vi "Error Handler.vi"(8 "error in (no error)":errorcluster, 9 "Error State":i32, 10 "Ignore Errors (Runtime)":i32[](array[numeric]), 11 "Queue In":refnum<queue>) -> (0 "dup error in":errorcluster, 3 "Queue Out":refnum<queue>)   [LabVIEW 2020, in "Enum Queue State Machine.lvlib"]
doc: "Process an error that occurred in the Event Handling Loop, either by ignoring it, or generating an \"Error\" message."
uses:
  Enum Queue State Machine.lvlib
  Controls/Enum Message.ctl
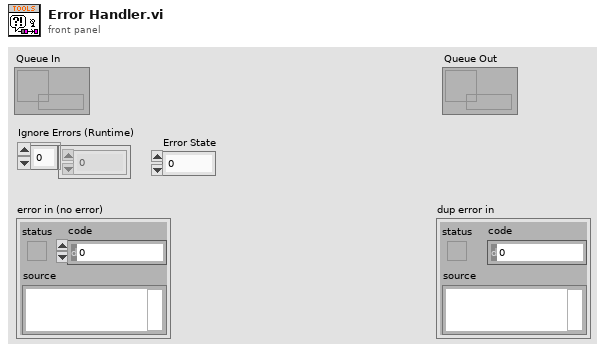
[diagram p1: front panel]
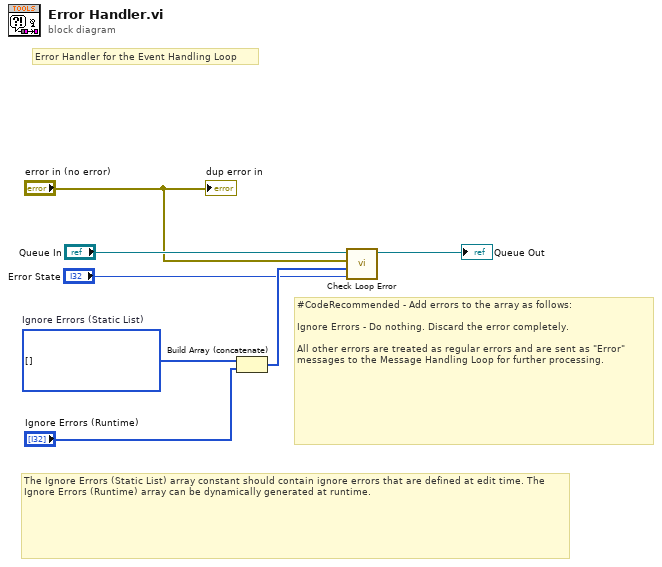
[diagram p0: block diagram]
diagram:
  w7 = i32[] []  # Ignore Errors (Static List)
  # "The Ignore Errors (Static List) array constant should contain ignore errors that are defined at edit time. The Ignore Errors (Runtime) array can be dynamically generated at runtime."
  # "#CodeRecommended - Add errors to the array as follows:\n\nIgnore Errors - Do nothing. Discard the error completely.\n\nAll other errors are treated as regular errors and are sent as \"Error\" messages to the Message Handling Loop for further processing."
  # "Error Handler for the Event Handling Loop"
  n1 = Build Array (concatenate)(w7, "Ignore Errors (Runtime)") -> (w3:i32[])
  n2 = call "Check Loop Error.vi"("Error State"="Error State", "Ignore Errors"=w3, "error to process"="error in (no error)", "Queue In"="Queue In") -> ("Queue Out"=→"Queue Out":refnum<queue>)  [unwired: 6 in, 1 out]
  "dup error in" <- "error in (no error)"
